vi "make_temp_api_vi_ref.vi"(6 "name of caller in":string, 9 "vi ref":refnum<vi>) -> (1 "api vi ref out":T1)   [LabVIEW 2015]
uses:
  cores/api_vi_ref.ctl
  <vilib>/GPower/String/Library/Typedefs/AllowedChars.ctl
  <vilib>/GPower/String/GPString.lvlib
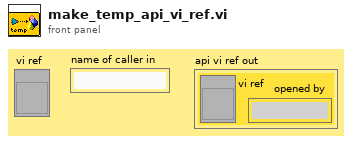
[diagram p1: front panel]
types:
  T1 = typedef "api_vi_ref.ctl" = cluster{"vi ref":refnum<vi>, "opened by":string}
  T2 = typedef "GPString.lvlib/AllowedChars.ctl" = enum16{"Any", "Alphanumeric", "Binary", "Hexadecimal", "Letters", "Lower case", "Numbers", "Octal", "Printable", "Upper case"}
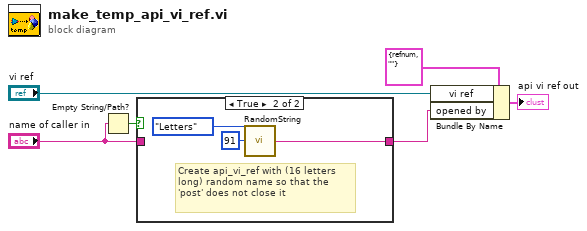
[diagram p0: block diagram]
diagram:
  n1 = Empty String/Path?(string/path="name of caller in") -> (empty?=w3:bool)
  n2 = case shown="True" w3 {
    tunnel: [w7 w8] -> w1
    tunnel: "name of caller in" -> [w7 _]
    frame False {
    }
    frame True {
      # "Create api_vi_ref with (16 letters long) random name so that the 'post' does not close it"
      n3 = call <vilib>:"RandomString.vi"("Randomness"=91, "Allowed characters"=AllowedChars."Letters") -> ("Random string"=w8:string)
    }
  }
  n4 = Bundle By Name(cluster=T1 {"vi ref"=refnum, "opened by"=""} ("api vi ref in"), "vi ref"="vi ref", "opened by"=w1) -> (→"api vi ref out":T1)
